vi "Read-Reg.vi"(8 "error in (no error)":errorcluster, 11 "Type-K-Thermocouple in":refnum<class "Pressure-Transducer.lvclass">) -> (0 "error out":errorcluster, 2 "Modbus-Reg":u16[](array[numeric]), 3 "Type-K-Thermocouple out":refnum<class "Pressure-Transducer.lvclass">)   [LabVIEW 2021, in "Pressure-Transducer.lvclass"]
uses:
  Pressure-Transducer.lvclass
  Modbus-Instr_class/Modbus-Instr.lvclass
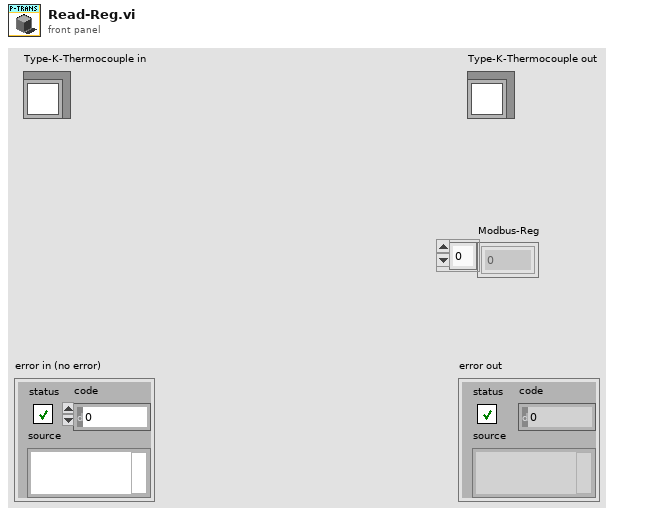
[diagram p1: front panel]
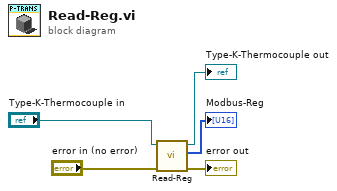
[diagram p0: block diagram]
diagram:
  n1 = call-parent "Read-Reg.vi"("error in (no error)"="error in (no error)", "Modbus-Instr in"="Type-K-Thermocouple in") -> ("error out"=→"error out":errorcluster, "Modbus-Reg"=→"Modbus-Reg":u16[], "Modbus-Instr out"=→"Type-K-Thermocouple out":refnum<class "Pressure-Transducer.lvclass">)  [unwired: 7 in]
